vi "PopulateMenu.vi"(0 "Enum":enum16{"Reset", "Populate"}(ring)=enum."Populate", 5 "error in":errorcluster) -> (6 "Left Menu":T1, 7 "Right Menu":T1, 8 "error out":errorcluster)   [LabVIEW 2016]
doc: "Populate or reset left and rigfht menu."
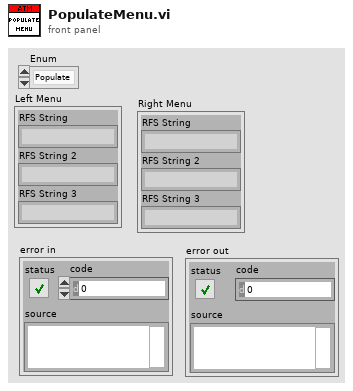
[diagram p1: front panel]
types:
  T1 = cluster{"RFS String":string, "RFS String 2":string, "RFS String 3":string}
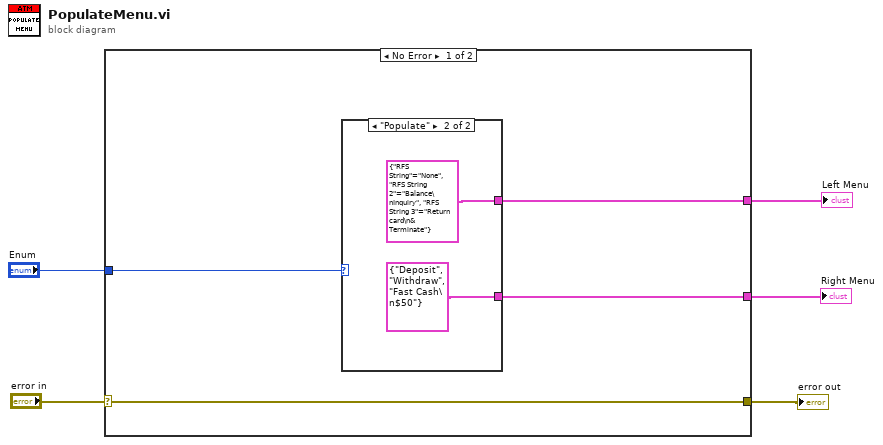
[diagram p0: block diagram]
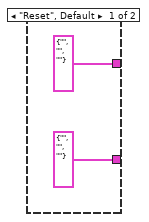
[diagram p2: hidden frame]
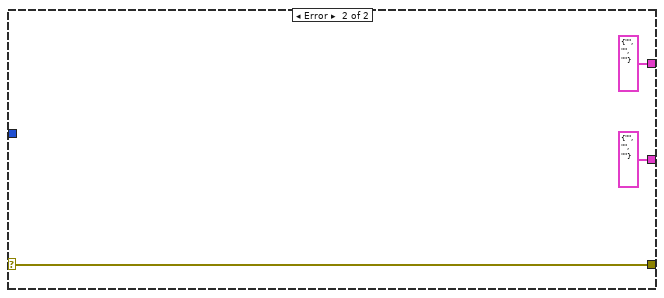
[diagram p3: hidden frame]
diagram:
  n1 = case shown="No Error" "error in" {
    selector: "error in" -> [w9 w16]
    tunnel: [w9 w16] -> w4
    tunnel: [w8 T1 {"RFS String"="", "RFS String 2"="", "RFS String 3"=""} ("Left Menu")] -> w3
    tunnel: [w7 T1 {"RFS String"="", "RFS String 2"="", "RFS String 3"=""} ("Right Menu")] -> w2
    tunnel: "Enum" -> [w6 _]
    frame No Error {
      n2 = case shown="\"Populate\"" w6 {
        tunnel: [T1 {"RFS String"="", "RFS String 2"="", "RFS String 3"=""} ("Left Menu") T1 {"RFS String"="None", "RFS String 2"="Balance\nInquiry", "RFS String 3"="Return card\n& Terminate"} ("Right Menu")] -> w8
        tunnel: [T1 {"RFS String"="", "RFS String 2"="", "RFS String 3"=""} ("Right Menu") T1 {"RFS String"="Deposit", "RFS String 2"="Withdraw", "RFS String 3"="Fast Cash\n$50"} ("Left Menu")] -> w7
        frame "Reset", Default {
        }
        frame "Populate" {
        }
      }
    }
    frame Error {
    }
  }
  "error out" <- w4
  "Right Menu" <- w2
  "Left Menu" <- w3
